vi "Configure Bitfile.vi"(0 "USRP RIO device":T1, 5 "which bitfile":string(combo)="Time", 11 "error in":errorcluster) -> (4 "USRP RIO device":T1, 6 "bitfile":path, 15 "error out":errorcluster)   [LabVIEW 2015]
uses:
  <vilib>/userdefined/Silver/nirio_resource_slv.ctl
  PPS_Global_Var.vi
  <vilib>/regexp/Match Regular Expression.xnode
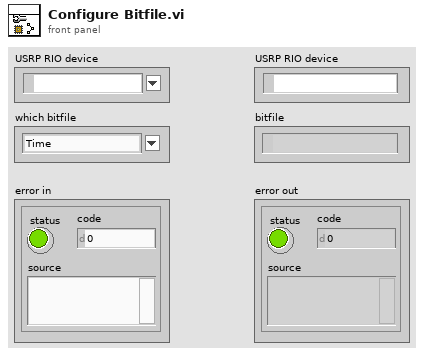
[diagram p1: front panel]
types:
  T1 = typedef "nirio_resource_slv.ctl" = tag
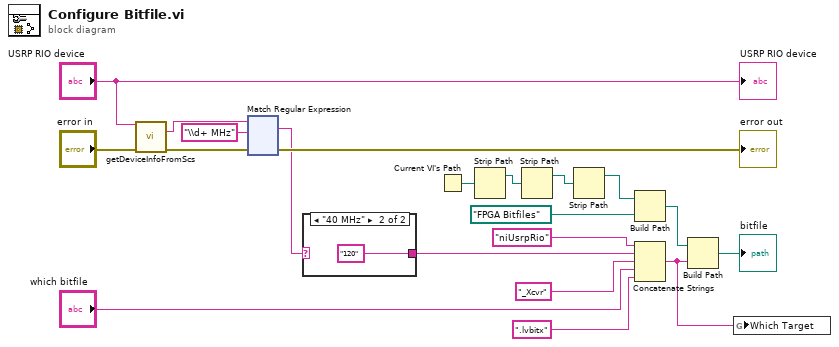
[diagram p0: block diagram]
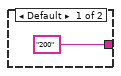
[diagram p2: hidden frame]
diagram:
  n1 = call <vilib>:"getDeviceInfoFromScs.vi"("rio device"="USRP RIO device", "error in"="error in") -> ("product name"=w5:string, "error out"=w6:errorcluster)  [unwired: 9 in, 3 out]
  n2 = xnode "Match Regular Expression"("input string"=w5, "regular expression"="\\d+ MHz", "error in"=w6) -> ("whole match"=w3:string, "error out"=→"error out":errorcluster)  [unwired: 3 in, 3 out]
  n3 = case shown="\"40 MHz\"" w3 {
    tunnel: ["200" ("format string") "120" ("format string")] -> w2
    frame Default {
    }
    frame "40 MHz" {
    }
  }
  n4 = Current VI's Path() -> (path=w20:path)
  n5 = Strip Path(path=w20) -> (stripped path=w17:path)  [unwired: 1 out]
  n6 = Strip Path(path=w17) -> (stripped path=w16:path)  [unwired: 1 out]
  n7 = Strip Path(path=w16) -> (stripped path=w15:path)  [unwired: 1 out]
  n8 = Build Path(base path=w15, name or relative path=path "FPGA Bitfiles") -> (appended path=w18:path)
  n9 = Concatenate Strings("niUsrpRio" ("format string"), w2, "_Xcvr" ("format string"), "which bitfile", ".lvbitx" ("format string")) -> (w1:string)
  n10 = Build Path(base path=w18, name or relative path=w1) -> (appended path=→"bitfile":path)
  n11 = global write "PPS_Global_Var.vi" "Which Target"(w1) -> ()
  "USRP RIO device" <- "USRP RIO device"
